vi "Assert MemberTable.vi"() -> ()   [LabVIEW 2015, in "Member_Actor.lvlib" / "TimeTable.lvclass"]
uses:
  TimeTable.lvclass
  TimeTable.lvclass/TimeTable.ctl
  Member_Actor.lvlib
panel:
  out "data":string[][](array[string])
  in  "SheetName(\"\")":string
  in  "Path":path
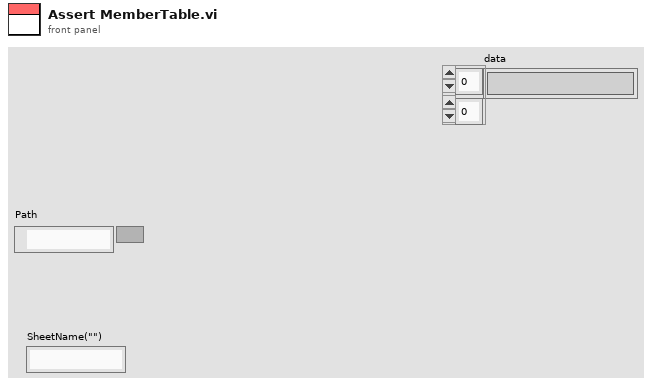
[diagram p1: front panel]
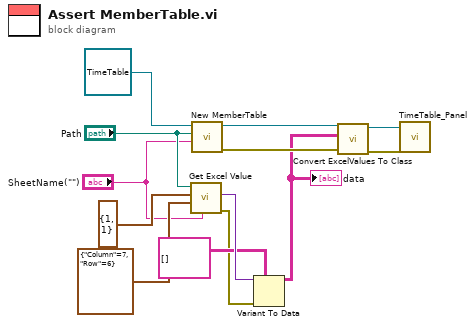
[diagram p0: block diagram]
diagram:
  n1 = call "Get Excel Value.vi"("SheetName(\"\")"="SheetName(\"\")", "End"=cluster{"Column":i32, "Row":i32} {"Column"=7, "Row"=6}, "Start"=cluster{"Column":i32, "Row":i32} {"Column"=1, "Row"=1}, "path"="Path") -> ("error out"=w2:errorcluster, "Excel_Value"=w4:variant)  [unwired: 6 in]
  n2 = call "New MemberTable.vi"("SheetName(\"\")"="SheetName(\"\")", "Path"="Path", "MemberTable in"=refnum<class "TimeTable.lvclass"> refnum) -> ("error out"=w11:errorcluster, "MemberTable out"=w12:refnum<class "TimeTable.lvclass">)  [unwired: 7 in]
  n3 = Variant To Data(error in=w2, type=string[][] [], Variant=w4) -> (data=w1:string[][])  [unwired: 1 out]
  "data" <- w1
  n4 = call "Convert ExcelValues To Class.vi"("error in (no error)"=w11, "Excel Value(\"\")"=w1, "MemberTable in"=w12) -> ("error out"=w9:errorcluster, "MemberTable out"=w10:refnum<class "TimeTable.lvclass">)  [unwired: 7 in]
  n5 = call "TimeTable_Panel.vi"("error in (no error)"=w9, "PanelController"=w10) -> ()  [unwired: 8 in, 2 out]
